vi "ModifyProjectDeployToGitCopy.vi"(11 "Arguments":string[](array[string])) -> (2 "Output error":string, 3 "Exit code":i32)   [LabVIEW 2021]
panel:
  out "error out":errorcluster
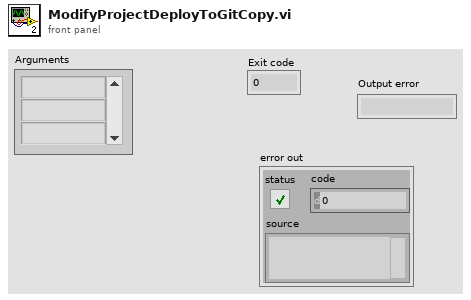
[diagram p1: front panel]
types:
  T1 = enum16{"open", "replace", "create", "open or create", "replace or create", "replace or create with confirmation"}
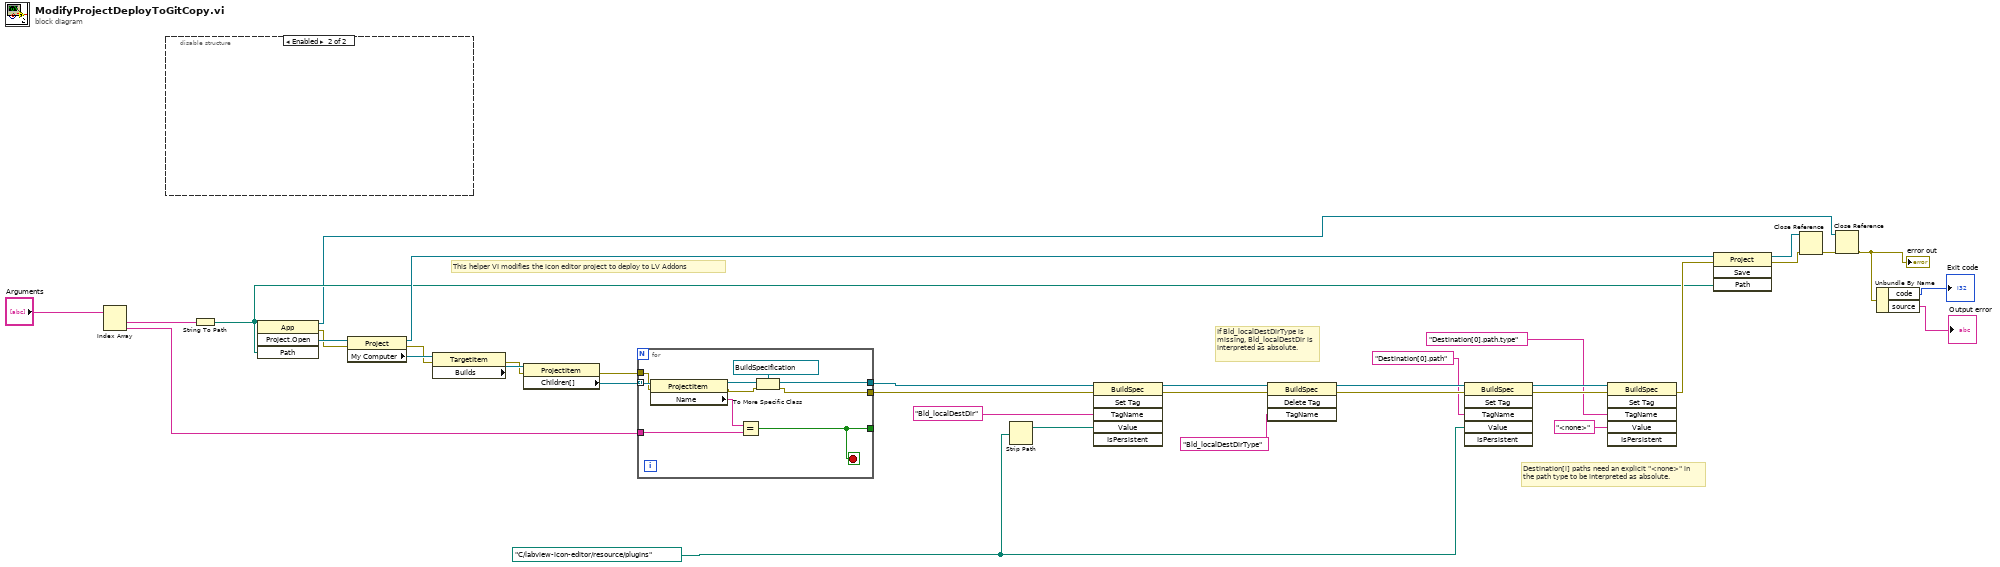
[diagram p0: block diagram]
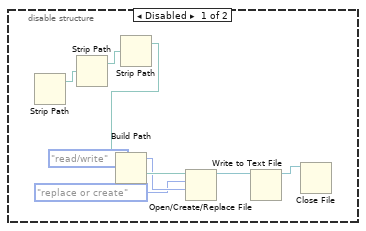
[diagram p2: hidden frame]
diagram:
  w1 = path "C:/labview-icon-editor/resource/plugins" ("path")
  # "Destination[i] paths need an explicit \"<none>\" in the path type to be interpreted as absolute."
  # "If Bld_localDestDirType is missing, Bld_localDestDir is interpreted as absolute."
  # "This helper VI modifies the icon editor project to deploy to LV Addons"
  n1 = Index Array(array="Arguments") -> (element #1=w10:string, element #2=w6:string)  [unwired: 2 in]
  n2 = disable-structure shown="Enabled" {
    frame Disabled {
      n3 = Strip Path() -> (stripped path=w42:path)  [unwired: 1 in, 1 out]
      n4 = Strip Path(path=w42) -> (stripped path=w41:path)  [unwired: 1 out]
      n5 = Strip Path(path=w41) -> (stripped path=w43:path)  [unwired: 1 out]
      n6 = Build Path(base path=w43) -> (appended path=w39:path)  [unwired: 1 in]
      n7 = Open/Create/Replace File(file path (use dialog)=w39, operation (0:open)=T1."replace or create", access (0:read/write)=enum16{"read/write", "read-only", "write-only"}."read/write") -> (refnum out=w40:refnum<file>)  [unwired: 3 in, 2 out]
      n8 = Write to Text File(file (use dialog)=w40) -> (refnum out=w44:refnum<file>)  [unwired: 3 in, 2 out]
      n9 = Close File(refnum=w44) -> ()  [unwired: 1 in, 2 out]
    }
    frame Enabled {
    }
  }
  n10 = String To Path(string=w10) -> (path=w9:path)
  n11 = invoke class="App" method="Project.Open"("Path"=w9) -> (reference out=w2:refnum<vi>, error out=w16:errorcluster, "Project:Open"=w31:refnum<vi>)  [unwired: 3 in, 1 out]
  n12 = property class="Project"(reference=w31, error in=w16) -> (reference out=w30:refnum<vi>, error out=w15:errorcluster, "My Computer"=w36:refnum<vi>)
  n13 = property class="TargetItem"(reference=w36, error in=w15) -> (error out=w14:errorcluster, "Builds"=w34:refnum<vi>)  [unwired: 1 out]
  n14 = property class="ProjectItem"(reference=w34, error in=w14) -> (error out=w13:errorcluster, "Children[]"=w35:refnum<vi>[])  [unwired: 1 out]
  n15 = for {
    tunnel: w35 -> [w54] mode=indexing
    tunnel: [w47] -> w33
    tunnel: w6 -> [w52]
    tunnel: [w51] -> _
    tunnel: [w48] -> w32
    tunnel: w13 -> [w45]
    stop <- w51 stop-if-true
    n16 = property class="ProjectItem"(reference=w54, error in=w45) -> (reference out=w49:refnum<vi>, error out=w50:errorcluster, "Name"=w53:string)
    n17 = Equal?(x=w53, y=w52) -> (x = y?=w51:bool)
    n18 = To More Specific Class(target class=refnum<vi> refnum ("Build Spec"), reference=w49, error in=w50) -> (specific class reference=w47:refnum<vi>, error out=w48:errorcluster)
  }
  n19 = Strip Path(path=w1) -> (stripped path=w17:path)  [unwired: 1 out]
  n20 = invoke class="BuildSpec" method="Set Tag"(reference=w33, error in=w32, "TagName"="Bld_localDestDir" ("Tag Name"), "Value"=w17) -> (reference out=w29:refnum<vi>, error out=w25:errorcluster)  [unwired: 2 in, 4 out]
  n21 = invoke class="BuildSpec" method="Delete Tag"(reference=w29, error in=w25, "TagName"="Bld_localDestDirType" ("Tag Name")) -> (reference out=w28:refnum<vi>, error out=w24:errorcluster)  [unwired: 1 in, 2 out]
  n22 = invoke class="BuildSpec" method="Set Tag"(reference=w28, error in=w24, "TagName"="Destination[0].path" ("format string"), "Value"=w1) -> (reference out=w23:refnum<vi>, error out=w22:errorcluster)  [unwired: 2 in, 4 out]
  n23 = invoke class="BuildSpec" method="Set Tag"(reference=w23, error in=w22, "TagName"="Destination[0].path.type" ("format string"), "Value"="<none>") -> (error out=w18:errorcluster)  [unwired: 2 in, 5 out]
  n24 = invoke class="Project" method="Save"(reference=w30, error in=w18, "Path"=w9) -> (reference out=w5:refnum<vi>, error out=w12:errorcluster)  [unwired: 1 in, 2 out]
  n25 = Close Reference(reference=w5, error in (no error)=w12) -> (error out=w4:errorcluster)
  n26 = Close Reference(reference=w2, error in (no error)=w4) -> (error out=w3:errorcluster)
  "error out" <- w3
  n27 = Unbundle By Name(w3) -> ("code"=→"Exit code":i32, "source"=→"Output error":string)
